vi "Init.vi"(8 "error in (no error)":errorcluster, 10 "Channel":i16, 11 "TrialBasedExperiment in":refnum<class "MatlabExperiment.lvclass">) -> (0 "error out":errorcluster, 3 "TrialBasedExperiment out":refnum<class "MatlabExperiment.lvclass">)   [LabVIEW 2012, in "AcquisitionCoreObjects.lvlib" / "MatlabExperiment.lvclass"]
uses:
  MatlabExperiment.lvclass
  TrialBasedExperimentObject/TrialBasedExperiment.lvclass
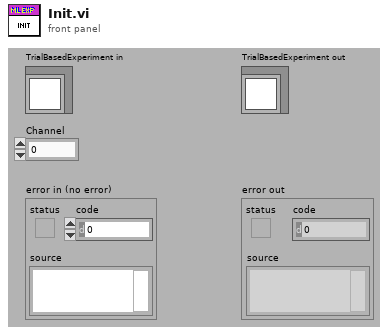
[diagram p1: front panel]
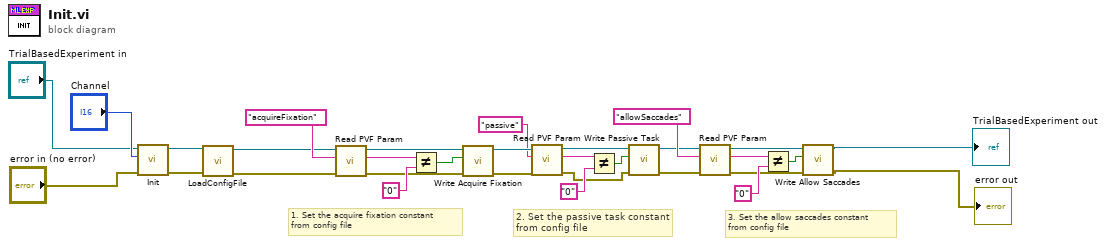
[diagram p0: block diagram]
diagram:
  # "3. Set the allow saccades constant\nfrom config file"
  # "2. Set the passive task constant\nfrom config file"
  # "1. Set the acquire fixation constant\nfrom config file"
  n1 = call-parent "Init.vi"("error in (no error)"="error in (no error)", "Channel"="Channel", "TrialBasedExperiment in"="TrialBasedExperiment in") -> ("error out"=w3:errorcluster, "TrialBasedExperiment out"=w4:refnum<class "MatlabExperiment.lvclass">)  [unwired: 7 in]
  n2 = call-dynamic "LoadConfigFile.vi"("error in (no error)"=w3, "MatlabExperiment in"=w4) -> ("error out"=w1:errorcluster, "MatlabExperiment out"=w2:refnum<class "MatlabExperiment.lvclass">)  [unwired: 8 in]
  n3 = call-dynamic "Read PVF Param.vi"("error in (no error)"=w1, "Param Name"="acquireFixation", "MatlabExperiment in"=w2) -> ("error out"=w26:errorcluster, "Param Value"=w30:string, "MatlabExperiment out"=w27:refnum<class "MatlabExperiment.lvclass">)  [unwired: 6 in]
  n4 = Not Equal?(x=w30, y="0") -> (x != y?=w28:bool)
  n5 = call-dynamic "Write Acquire Fixation.vi"("error in (no error)"=w26, "Acquire Fixation"=w28, "TrialBasedExperiment in"=w27) -> ("error out"=w25:errorcluster, "TrialBasedExperiment out"=w24:refnum<class "MatlabExperiment.lvclass">)  [unwired: 7 in]
  n6 = call-dynamic "Read PVF Param.vi"("error in (no error)"=w25, "Param Name"="passive", "MatlabExperiment in"=w24) -> ("error out"=w20:errorcluster, "Param Value"=w21:string, "MatlabExperiment out"=w19:refnum<class "MatlabExperiment.lvclass">)  [unwired: 6 in]
  n7 = Not Equal?(x=w21, y="0") -> (x != y?=w18:bool)
  n8 = call-dynamic "Write Passive Task.vi"("error in (no error)"=w20, "Passive Task"=w18, "TrialBasedExperiment in"=w19) -> ("error out"=w15:errorcluster, "TrialBasedExperiment out"=w16:refnum<class "MatlabExperiment.lvclass">)  [unwired: 7 in]
  n9 = call-dynamic "Read PVF Param.vi"("error in (no error)"=w15, "Param Name"="allowSaccades", "MatlabExperiment in"=w16) -> ("error out"=w12:errorcluster, "Param Value"=w13:string, "MatlabExperiment out"=w11:refnum<class "MatlabExperiment.lvclass">)  [unwired: 6 in]
  n10 = Not Equal?(x=w13, y="0") -> (x != y?=w10:bool)
  n11 = call-dynamic "Write Allow Saccades.vi"("error in (no error)"=w12, "Allow Saccades"=w10, "TrialBasedExperiment in"=w11) -> ("error out"=→"error out":errorcluster, "TrialBasedExperiment out"=→"TrialBasedExperiment out":refnum<class "MatlabExperiment.lvclass">)  [unwired: 7 in]
